vi "Property Dialog.vi"(6 "Control Ref Queue":T29, 7 "Data":refnum<class "3D Plot Datatype.lvclass">[](array[class]), 8 "error in (no error)":errorcluster, 9 "Object Cluster In":T28, 11 "3D Bar in":refnum<class "3D Bar.lvclass">) -> (0 "error out":errorcluster, 1 "Object Cluster Out":T28, 3 "3D Bar out":refnum<class "3D Bar.lvclass">, 4 "Cancel?":bool)   [LabVIEW 2020, in "3D Bar.lvclass"]
uses:
  <vilib>/Math Plots/3D Math Plots/3D Bar/3D Bar/3D Bar.lvclass
  e:/builds/penguin/labview/branches/2020/dev/dist/vi.lib/Math Plots/3D Math Plots/3D Plot/3D Plot/3D Plot.lvclass
  <vilib>/Math Plots/3D Math Plots/3D Plot/Action String/3DMathPlot Ctrl Act Queue.ctl
  <vilib>/Math Plots/3D Math Plots/3D Plot/Action String/3DMathPlot Ctrl Act Cluster.ctl
  <vilib>/Math Plots/3D Math Plots/3D Plot/Action String/3DMathPlot State Class.ctl
  <vilib>/Math Plots/3D Math Plots/3D Plot/3D Plot/Typedef/Object Cluster.ctl
  <vilib>/Math Plots/3D Math Plots/3D Plot/3D Plot Datatype/3D Plot Datatype.lvclass
  <vilib>/Math Plots/3D Math Plots/3D Bar/3D Bar/Typedef/3D Bar Property Array.ctl
  <vilib>/Math Plots/3D Math Plots/3D Bar/3D Bar/Typedef/3D Bar Property.ctl
  <vilib>/Math Plots/3D Math Plots/3D Plot/3D Plot/Typedef/Line Type.ctl
  <vilib>/Math Plots/3D Math Plots/3D Plot/3D Plot/Typedef/Cursor Property Array.ctl
  <vilib>/Math Plots/3D Math Plots/3D Plot/3D Plot/Typedef/Cursor Property.ctl
  <vilib>/Math Plots/3D Math Plots/3D Plot/3D Plot/Typedef/Cursor Position.ctl
  <vilib>/Math Plots/3D Math Plots/3D Plot/3D Plot/Typedef/Cursor Point.ctl
  <vilib>/Math Plots/3D Math Plots/3D Plot/3D Plot/Typedef/Sprite Type.ctl
  <vilib>/Math Plots/3D Math Plots/3D Plot/3D Plot/Typedef/Cursor Line.ctl
  <vilib>/Math Plots/3D Math Plots/3D Plot/3D Plot/Typedef/Cursor Plane.ctl
  <vilib>/Math Plots/3D Math Plots/3D Plot/3D Plot/Typedef/Cursor Text.ctl
  <vilib>/Math Plots/3D Math Plots/3D Plot/3D Plot/Typedef/Format Property.ctl
  <vilib>/Math Plots/3D Math Plots/3D Plot/3D Plot/Typedef/Value Pair Property.ctl
  <vilib>/Math Plots/3D Math Plots/3D Plot/3D Plot/Typedef/Value Pair Cluster.ctl
  <vilib>/Math Plots/3D Math Plots/3D Plot/3D Plot/Typedef/Axis Property.ctl
  <vilib>/Math Plots/3D Math Plots/3D Plot/3D Plot/Typedef/Caption Property.ctl
  <vilib>/Math Plots/3D Math Plots/3D Plot/3D Plot/Typedef/Label Property.ctl
  <vilib>/Math Plots/3D Math Plots/3D Plot/3D Plot/Typedef/Range Property.ctl
  <vilib>/Math Plots/3D Math Plots/3D Plot/3D Plot/Typedef/Range Clusters.ctl
  <vilib>/Math Plots/3D Math Plots/3D Plot/3D Plot/Typedef/Grid Property.ctl
  <vilib>/Math Plots/3D Math Plots/3D Plot/3D Plot/Typedef/Tick Property.ctl
  <vilib>/Math Plots/3D Math Plots/3D Plot/3D Plot/Typedef/Light Property.ctl
  <vilib>/Math Plots/3D Math Plots/3D Plot/3D Plot/Typedef/Light Specific.ctl
  <vilib>/Math Plots/3D Math Plots/3D Plot/3D Plot/Typedef/Graph Property.ctl
  <vilib>/Math Plots/3D Math Plots/3D Plot/3D Plot/Typedef/General Property.ctl
  <vilib>/Math Plots/3D Math Plots/3D Plot/3D Plot/Typedef/View Property.ctl
  <vilib>/Math Plots/3D Math Plots/3D Plot/3D Plot/Typedef/Grid Plane.ctl
  <vilib>/Math Plots/3D Math Plots/3D Plot/3D Plot/Typedef/Temp Scene State.ctl
  <vilib>/Math Plots/3D Math Plots/3D Plot/3D Plot/Typedef/Temp Scene Data Action.ctl
  <vilib>/Math Plots/3D Math Plots/3D Bar/3D Bar/3D Bar.lvclass/3D Bar.ctl
  <vilib>/Math Plots/3D Math Plots/3D Plot/3D Plot/3D Plot.lvclass
panel:
  in  "Graph Property":T1
  in  "Light Property":T5
  in  "Axis Property":T7
  in  "Value Pair Property":T14
  in  "Format Property":T16
  in  "Cursor Property Array":T17
  in  "3D Bar Property Array":T26
  in  "Dialog Tab":enum32{"UI", "Input & Output"}(tab)
  in  "Cancel":bool
  in  "Help":bool
  in  "OK":bool
  in  "Page List":i32(listbox) caption="Page list"
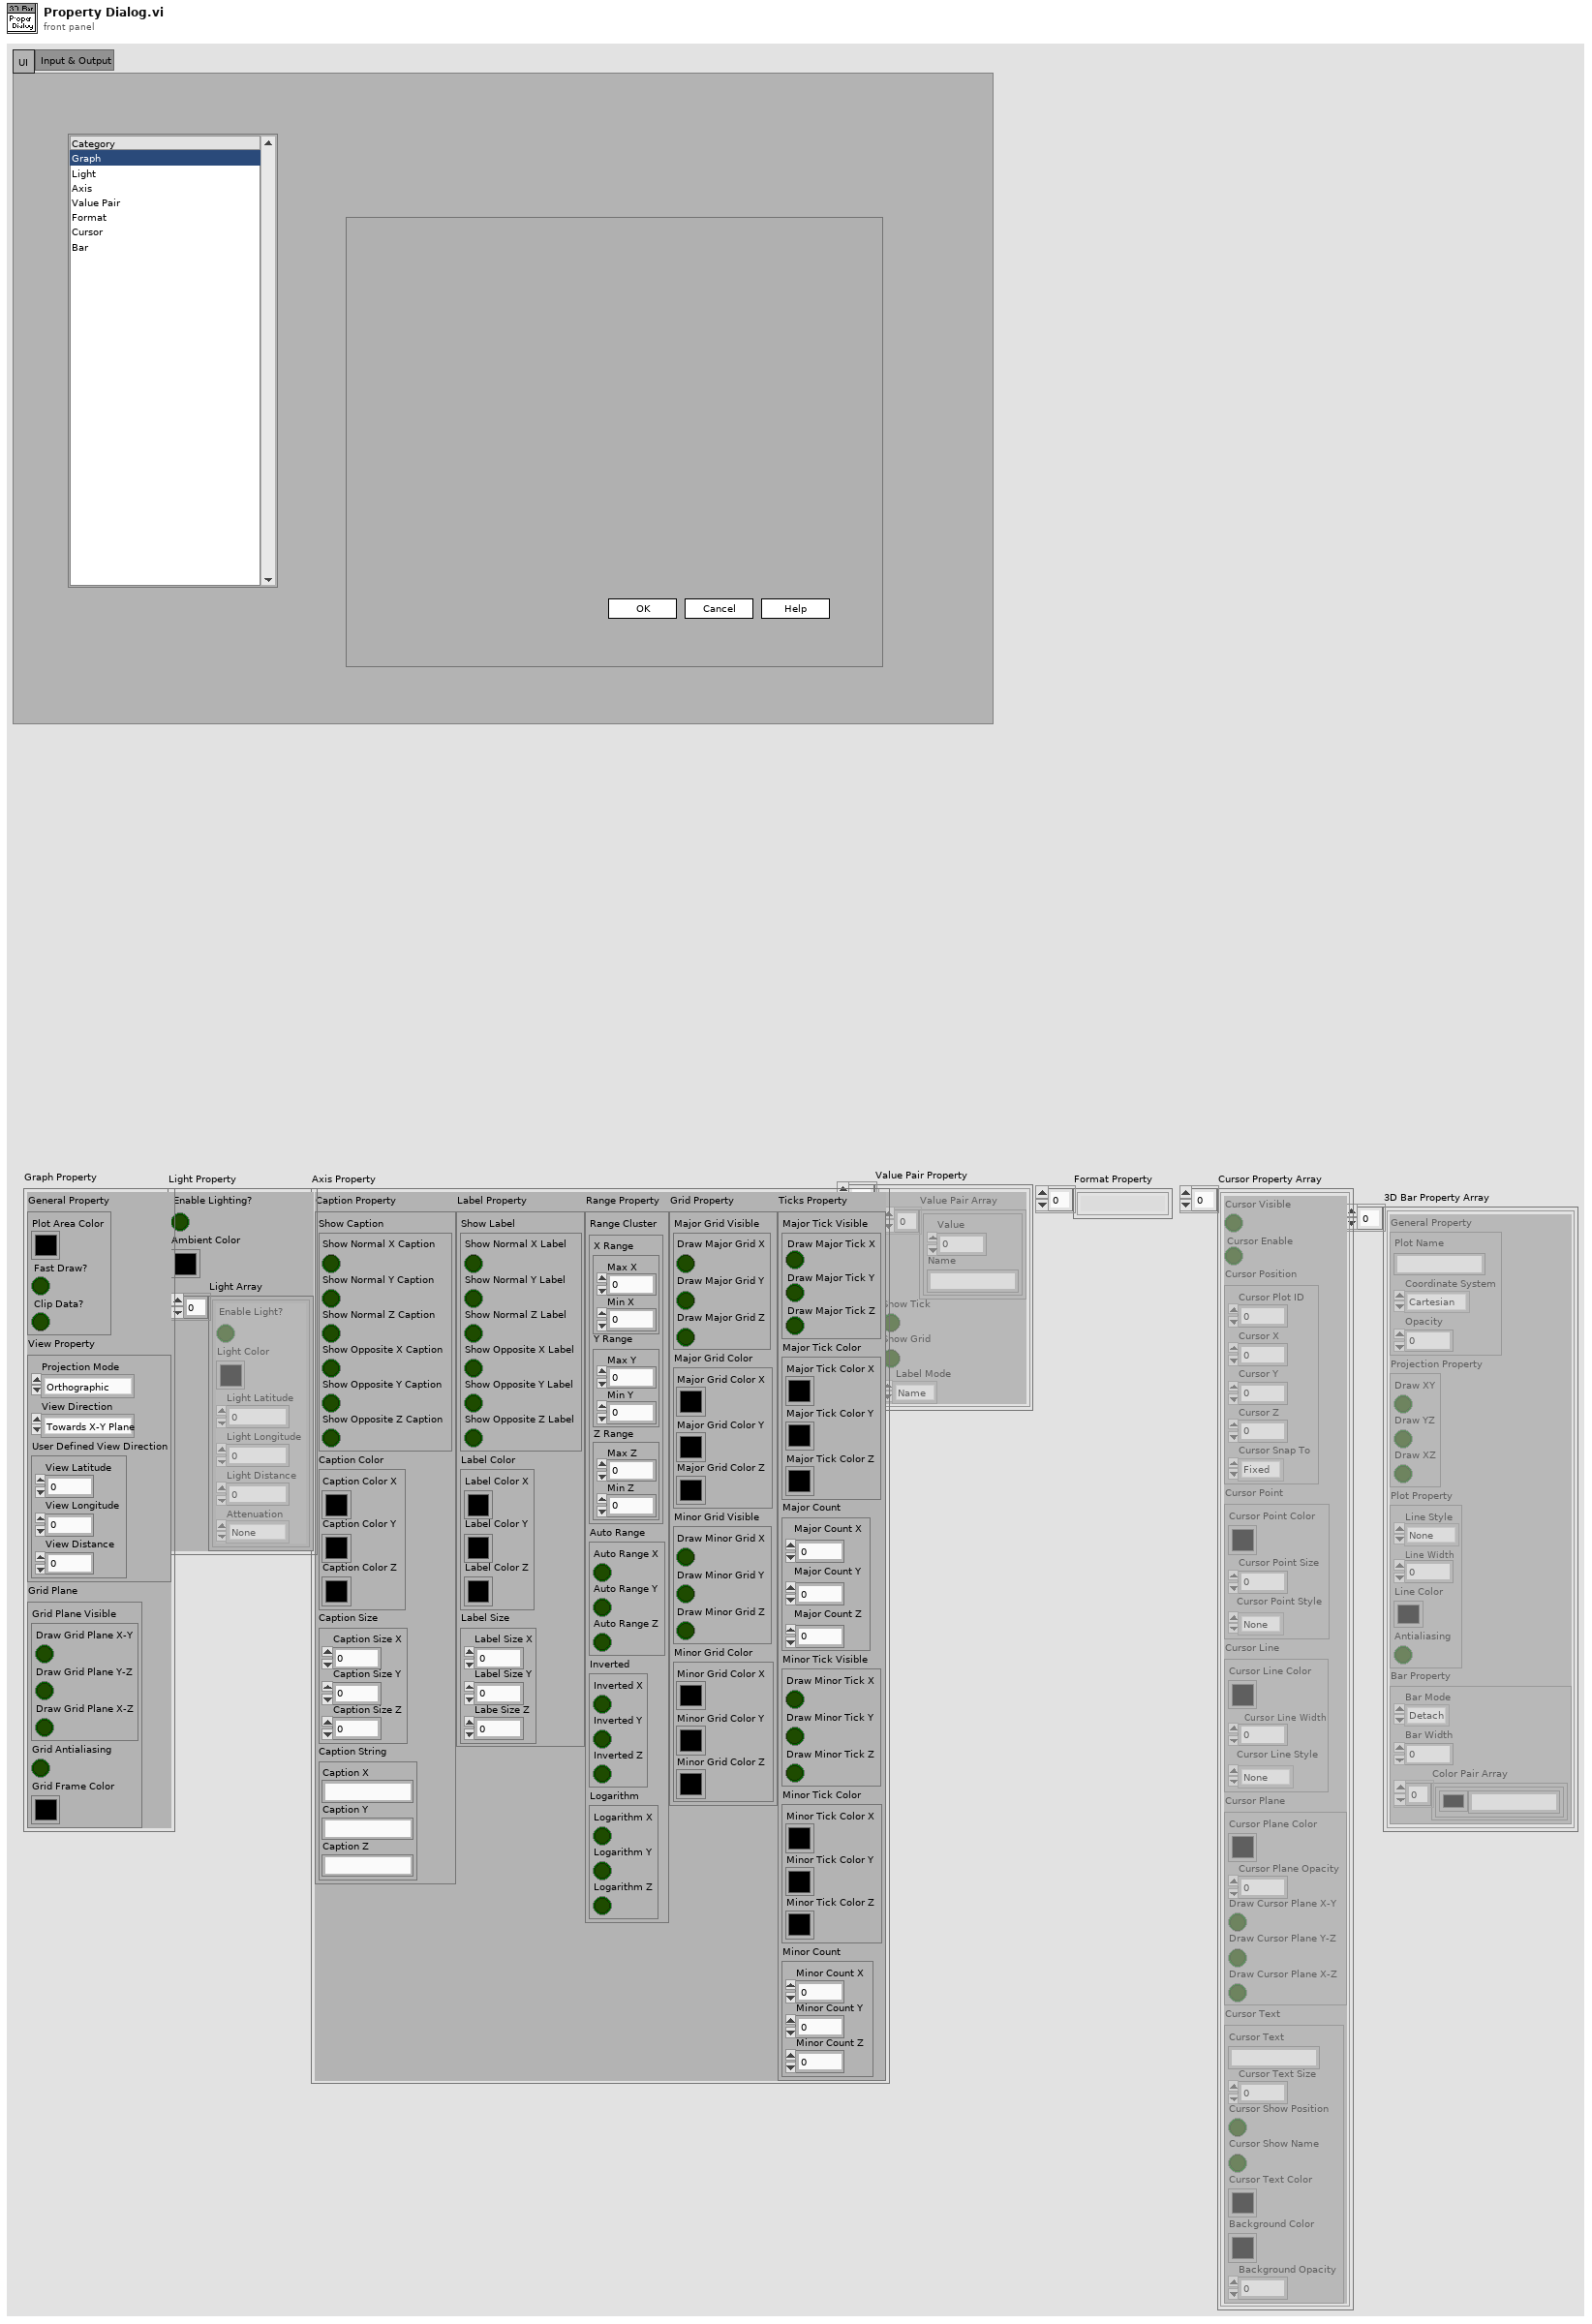
[diagram p1: front panel]
types:
  T1 = typedef "3D Plot.lvclass/Graph Property.ctl" = cluster{"General Property":T2, "View Property":T3, "Grid Plane":T4}
  T2 = typedef "3D Plot.lvclass/General Property.ctl" = cluster{"Plot Area Color":u32, "Fast Draw?":bool, "Clip Data?":bool}
  T3 = typedef "3D Plot.lvclass/View Property.ctl" = cluster{"Projection Mode":enum16{"Orthographic", "Perspective"}, "View Direction":enum32{"Towards X-Y Plane", "Towards X-Z Plane", "Towards Y-Z Plane", "User Defined"}, "User Defined View Direction":cluster{"View Latitude":sgl, "View Longitude":sgl, "View Distance":sgl}}
  T4 = typedef "3D Plot.lvclass/Grid Plane.ctl" = cluster{"Grid Plane Visible":cluster{"Draw Grid Plane X-Y":bool, "Draw Grid Plane Y-Z":bool, "Draw Grid Plane X-Z":bool}, "Grid Antialiasing":bool, "Grid Frame Color":u32}
  T5 = typedef "3D Plot.lvclass/Light Property.ctl" = cluster{"Enable Lighting?":bool, "Ambient Color":u32, "Light Array":T6[]}
  T6 = typedef "3D Plot.lvclass/Light Specific.ctl" = cluster{"Enable Light?":bool, "Light Color":u32, "Light Latitude":sgl, "Light Longitude":sgl, "Light Distance":sgl, "Attenuation":enum16{"None", "Linear", "Quadratic"}}
  T7 = typedef "3D Plot.lvclass/Axis Property.ctl" = cluster{"Caption Property":T8, "Label Property":T9, "Range Property":T10, "Grid Property":T12, "Ticks Property":T13}
  T8 = typedef "3D Plot.lvclass/Caption Property.ctl" = cluster{"Show Caption":cluster{"Show Normal X Caption":bool, "Show Normal Y Caption":bool, "Show Normal Z Caption":bool, "Show Opposite X Caption":bool, "Show Opposite Y Caption":bool, "Show Opposite Z Caption":bool}, "Caption Color":cluster{"Caption Color X":u32, "Caption Color Y":u32, "Caption Color Z":u32}, "Caption Size":cluster{"Caption Size X":u16, "Caption Size Y":u16, "Caption Size Z":u16}, "Caption String":cluster{"Caption X":string, "Caption Y":string, "Caption Z ":string}}
  T9 = typedef "3D Plot.lvclass/Label Property.ctl" = cluster{"Show Label":cluster{"Show Normal X Label":bool, "Show Normal Y Label":bool, "Show Normal Z Label":bool, "Show Opposite X Label":bool, "Show Opposite Y Label":bool, "Show Opposite Z Label":bool}, "Label Color":cluster{"Label Color X":u32, "Label Color Y":u32, "Label Color Z":u32}, "Label Size":cluster{"Label Size X":u16, "Label Size Y":u16, "Labe Size Z":u16}}
  T10 = typedef "3D Plot.lvclass/Range Property.ctl" = cluster{"Range Cluster":T11, "Auto Range":cluster{"Auto Range X":bool, "Auto Range Y":bool, "Auto Range Z":bool}, "Inverted":cluster{"Inverted X":bool, "Inverted Y":bool, "Inverted Z":bool}, "Logarithm":cluster{"Logarithm X":bool, "Logarithm Y":bool, "Logarithm Z":bool}}
  T11 = typedef "3D Plot.lvclass/Range Clusters.ctl" = cluster{"X Range":cluster{"Max X":sgl, "Min X":sgl}, "Y Range":cluster{"Max Y":sgl, "Min Y":sgl}, "Z Range":cluster{"Max Z":sgl, "Min Z":sgl}}
  T12 = typedef "3D Plot.lvclass/Grid Property.ctl" = cluster{"Major Grid Visible":cluster{"Draw Major Grid X":bool, "Draw Major Grid Y":bool, "Draw Major Grid Z":bool}, "Major Grid Color":cluster{"Major Grid Color X":u32, "Major Grid Color Y":u32, "Major Grid Color Z":u32}, "Minor Grid Visible":cluster{"Draw Minor Grid X":bool, "Draw Minor Grid Y":bool, "Draw Minor Grid Z":bool}, "Minor Grid Color":cluster{"Minor Grid Color X":u32, "Minor Grid Color Y":u32, "Minor Grid Color Z":u32}}
  T13 = typedef "3D Plot.lvclass/Tick Property.ctl" = cluster{"Major Tick Visible":cluster{"Draw Major Tick X":bool, "Draw Major Tick Y":bool, "Draw Major Tick Z":bool}, "Major Tick Color":cluster{"Major Tick Color X":u32, "Major Tick Color Y":u32, "Major Tick Color Z":u32}, "Major Count":cluster{"Major Count X":u16, "Major Count Y":u16, "Major Count Z":u16}, "Minor Tick Visible":cluster{"Draw Minor Tick X":bool, "Draw Minor Tick Y":bool, "Draw Minor Tick Z":bool}, "Minor Tick Color":cluster{"Minor Tick Color X":u32, "Minor Tick Color Y":u32, "Minor Tick Color Z":u32}, "Minor Count":cluster{"Minor Count X":u16, "Minor Count Y":u16, "Minor Count Z":u16}}
  T14 = typedef "3D Plot.lvclass/Value Pair Property.ctl" = T15[]
  T15 = typedef "3D Plot.lvclass/Value Pair Cluster.ctl" = cluster{"Value Pair Array":cluster{"Value":sgl, "Name":string}[], "Show Tick":bool, "Show Grid":bool, " Label Mode":enum16{"Name", "Value", "None"}}
  T16 = typedef "3D Plot.lvclass/Format Property.ctl" = string[]
  T17 = typedef "3D Plot.lvclass/Cursor Property Array.ctl" = T18[]
  T18 = typedef "3D Plot.lvclass/Cursor Property.ctl" = cluster{"Cursor Visible":bool, "Cursor Enable":bool, "Cursor Position":T19, "Cursor Point":T20, "Cursor Line":T22, "Cursor Plane":T24, "Cursor Text":T25}
  T19 = typedef "3D Plot.lvclass/Cursor Position.ctl" = cluster{"Cursor Plot ID":i32, "Cursor X":sgl, "Cursor Y":sgl, "Cursor Z":sgl, "Cursor Snap To":enum16{"Fixed", "Nearest Plot", "Snap to Plot"}}
  T20 = typedef "3D Plot.lvclass/Cursor Point.ctl" = cluster{"Cursor Point Color":u32, "Cursor Point Size":sgl, "Cursor Point Style":T21}
  T21 = typedef "3D Plot.lvclass/Sprite Type.ctl" = enum16{"None", "Empty Square", "Solid Square", "Empty Diamond", "Solid Diamond", "Empty Circle", "Solid Circle", "Asterisk", "Bold X", "Wireframe Sphere", "Solid Sphere", "Wireframe Cube", "Solid Cube"}
  T22 = typedef "3D Plot.lvclass/Cursor Line.ctl" = cluster{"Cursor Line Color":u32, "Cursor Line Width":sgl, "Cursor Line Style":T23}
  T23 = typedef "3D Plot.lvclass/Line Type.ctl" = enum16{"None", "Solid", "Dash", "Dot", "Dash Dot"}
  T24 = typedef "3D Plot.lvclass/Cursor Plane.ctl" = cluster{"Cursor Plane Color":u32, "Cursor Plane Opacity":sgl, "Draw Cursor Plane X-Z":bool, "Draw Cursor Plane Y-Z":bool, "Draw Cursor Plane X-Y":bool}
  T25 = typedef "3D Plot.lvclass/Cursor Text.ctl" = cluster{"Cursor Text":string, "Cursor Text Size":u16, "Cursor Show Position":bool, "Cursor Show Name":bool, "Cursor Text Color":u32, "Background Color":u32, "Background Opacity":sgl}
  T26 = typedef "3D Bar.lvclass/3D Bar Property Array.ctl" = T27[]
  T27 = typedef "3D Bar.lvclass/3D Bar Property.ctl" = cluster{"General Property":cluster{"Plot Name":string, "Coordinate System":enum16{"Cartesian", "Cylindrical", "Spherical"}, "Opacity":sgl}, "Projection Property":cluster{"Draw XY":bool, "Draw YZ":bool, "Draw XZ":bool}, "Plot Property":cluster{"Line Style":T23, "Line Width":sgl, "Line Color":u32, "Antialiasing":bool}, "Bar Property":cluster{"Bar Mode":enum16{"Detach", "Group", "Stack"}, "Bar Width":sgl, "Color Pair Array":cluster{"Color":u32, "String":string}[]}}
  T28 = typedef "3D Plot.lvclass/Object Cluster.ctl" = cluster{"Root Scene Object":refnum<vi>, "Fast Root Scene Object":refnum<vi>}
  T29 = typedef "3DMathPlot Ctrl Act Queue.ctl" = refnum<queue>
  T30 = typedef "3D Plot.lvclass/Temp Scene State.ctl" = enum16{"Create", "Update Scene", "Get Plot Representation", "Destory"}
  T31 = typedef "3D Plot.lvclass/Temp Scene Data Action.ctl" = enum16{"Data Class", "Property Class", "Object Cluster", "Control Queue"}
  T32 = typedef "3D Plot.lvclass/Property Cluster.ctl" = cluster{"Graph Property":T1, "Light Property":T5, "Axis Property":T7, "Value Pair Property":T14, "Format Property":T16, "Cursor Property Array":T17, "Appearance Property":T33}
  T33 = typedef "3D Plot.lvclass/Apearance Property.ctl" = cluster{"Visibility":T34, "Active Index":cluster{"Active Plot":i32, "Active Cursor":i32, "Active Axis":enum16{"X-axis", "Y-axis", "Z-axis"}, "Active Value Pair":enum16{"X-axis", "Y-axis", "Z-axis"}, "Active Light":enum16{"Light 0", "Light 1", "Light 2", "Light 3"}}, "Backup Data":cluster{"Plot Name":string[]}}
  T34 = typedef "3D Plot.lvclass/Item Visibility.ctl" = cluster{"Projection Palette":bool, "Color Ramp Palette":bool}
  T35 = enum32{"Bad", "Idle", "Run top level", "Running"}[]
  T36 = enum32{"Bad", "Idle", "Run top level", "Running"}
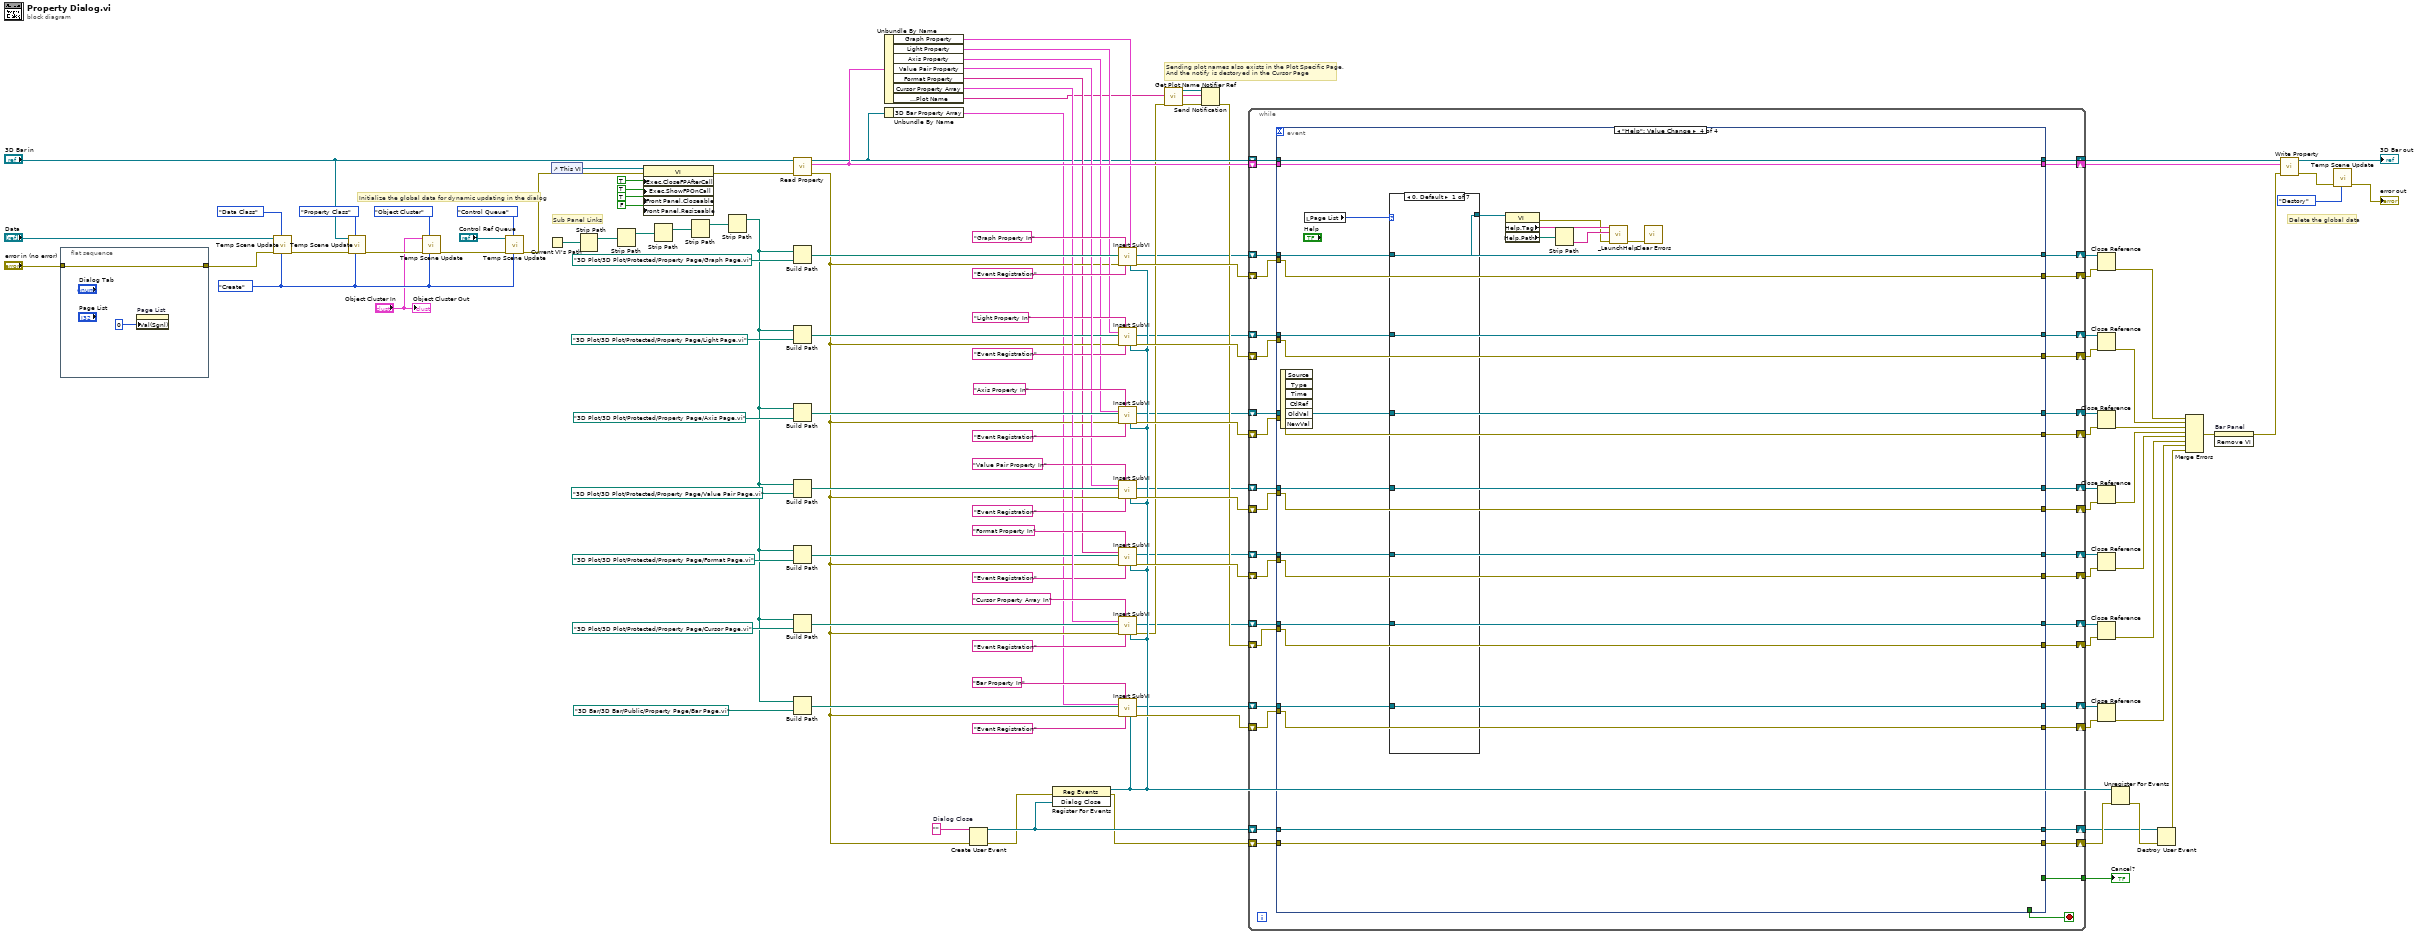
[diagram p0: block diagram]
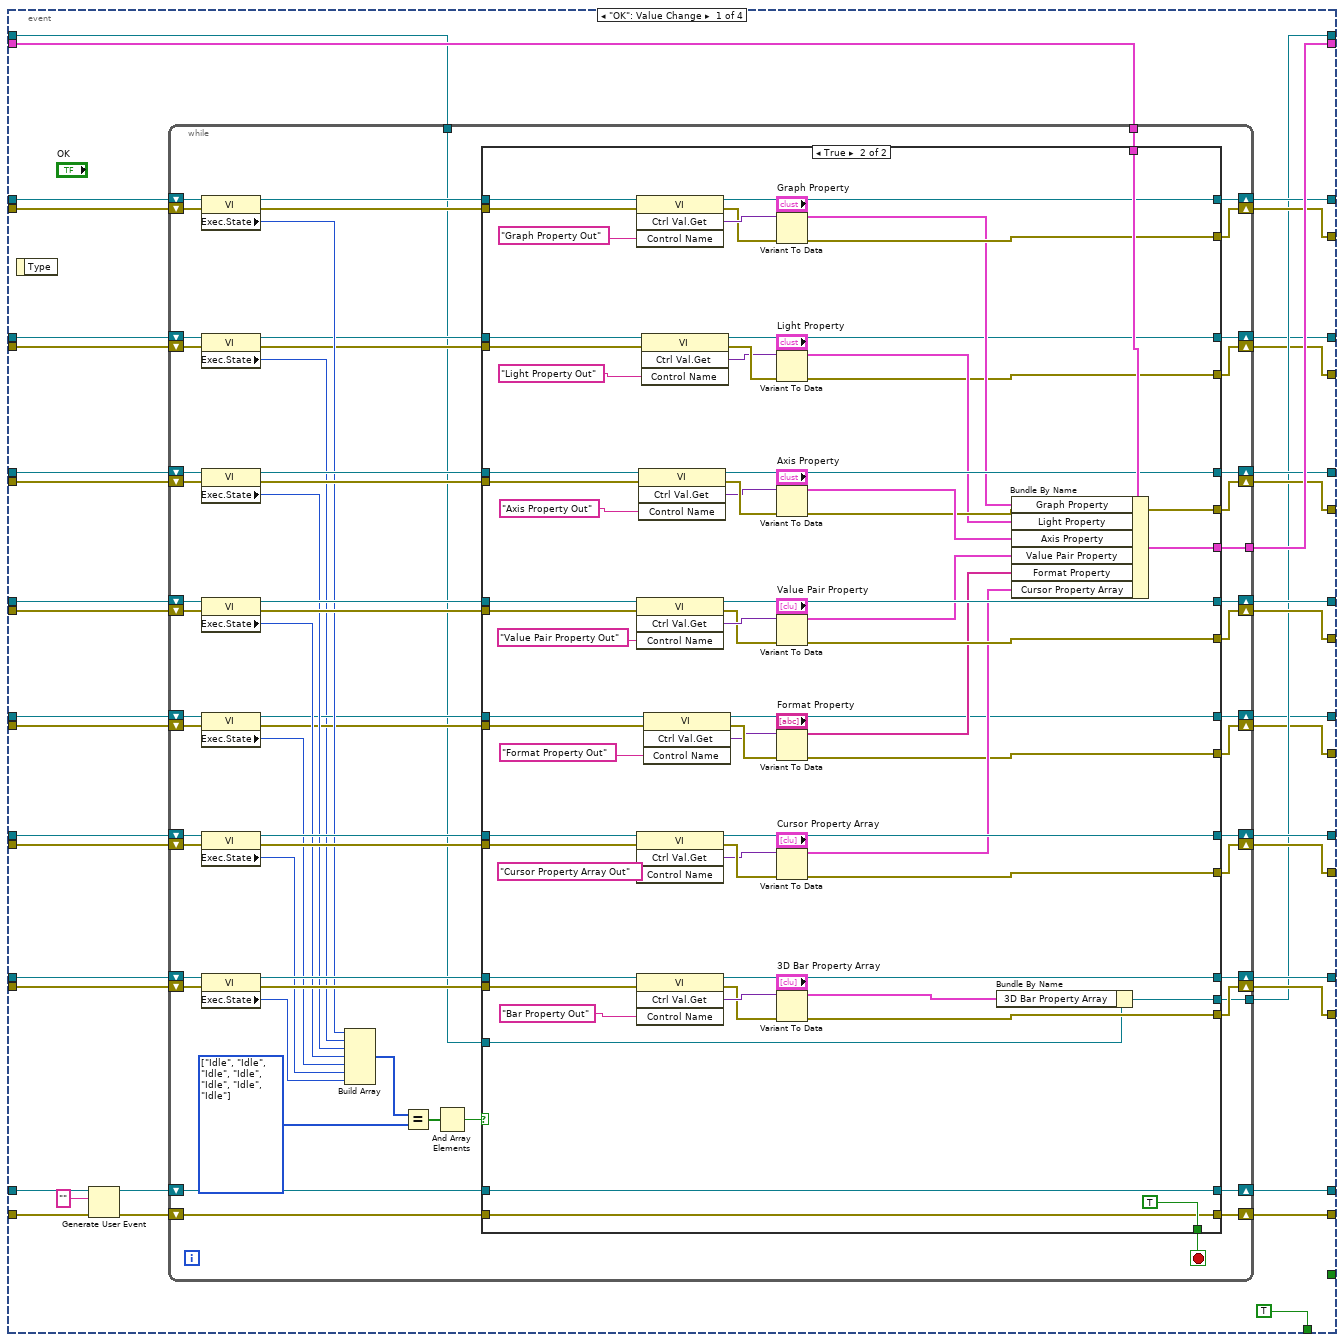
[diagram p2: hidden frame]
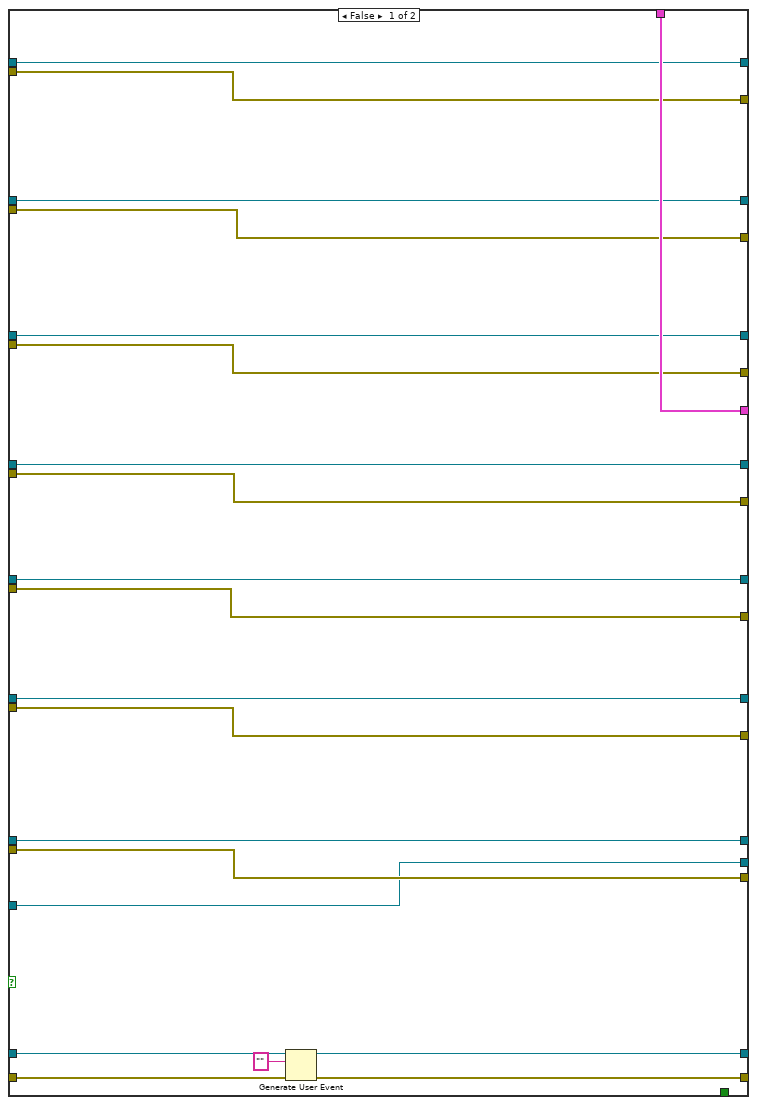
[diagram p3: hidden frame]
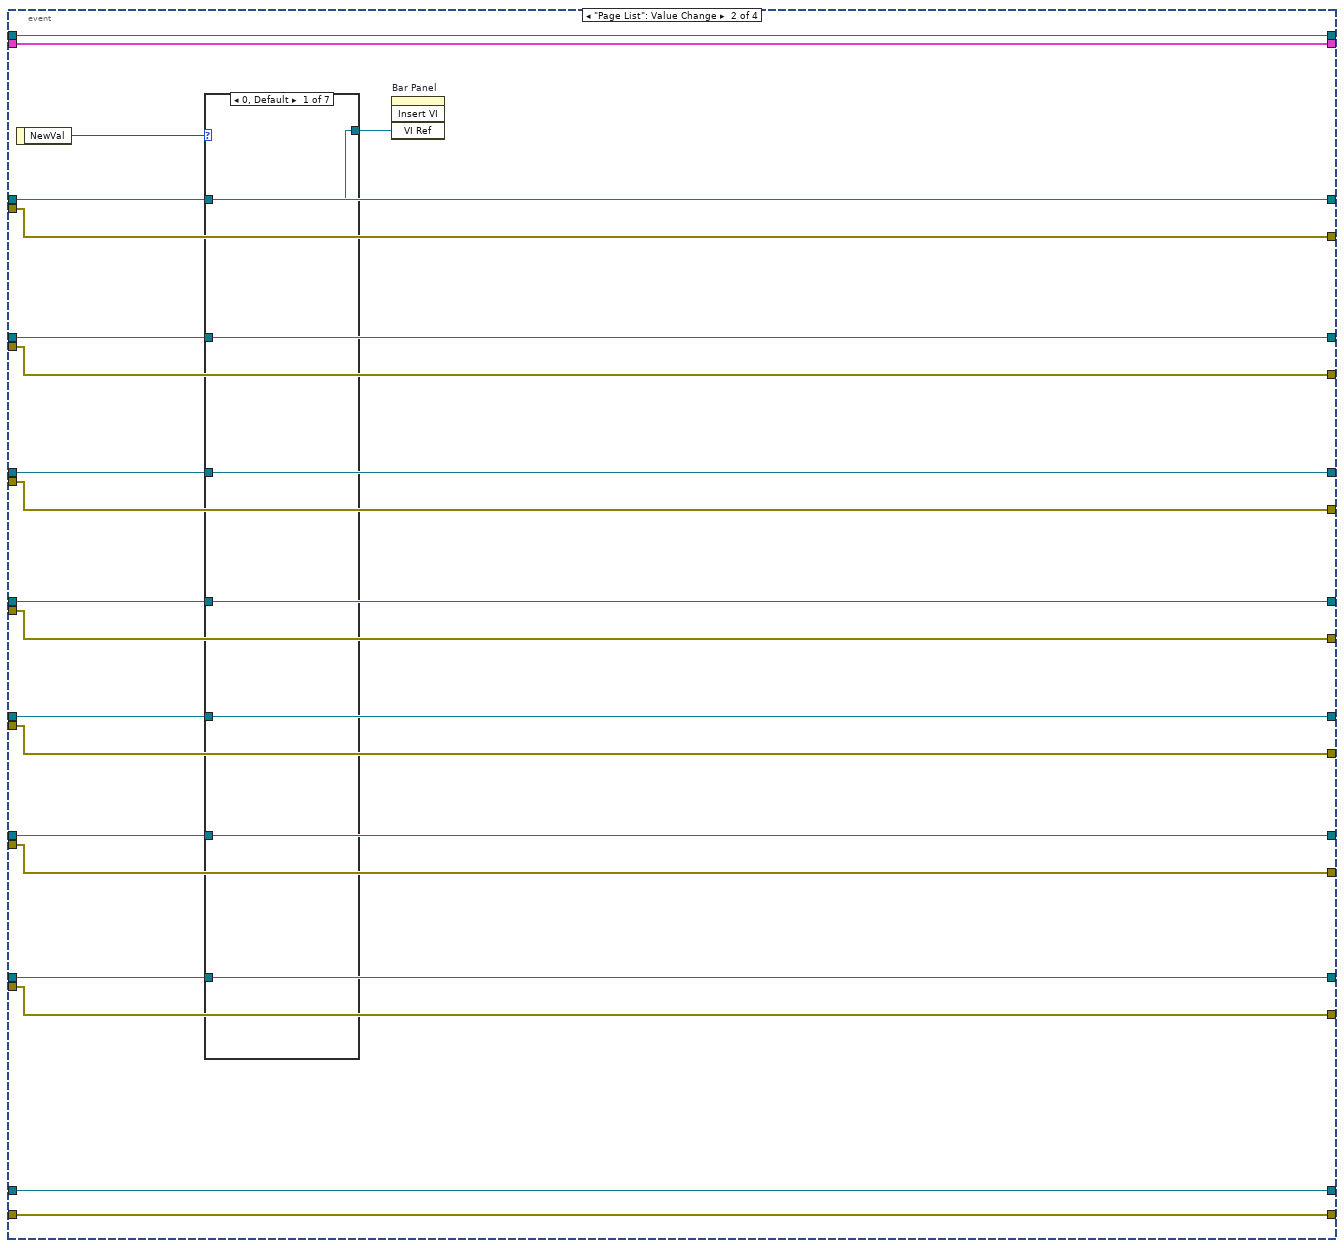
[diagram p4: hidden frame]
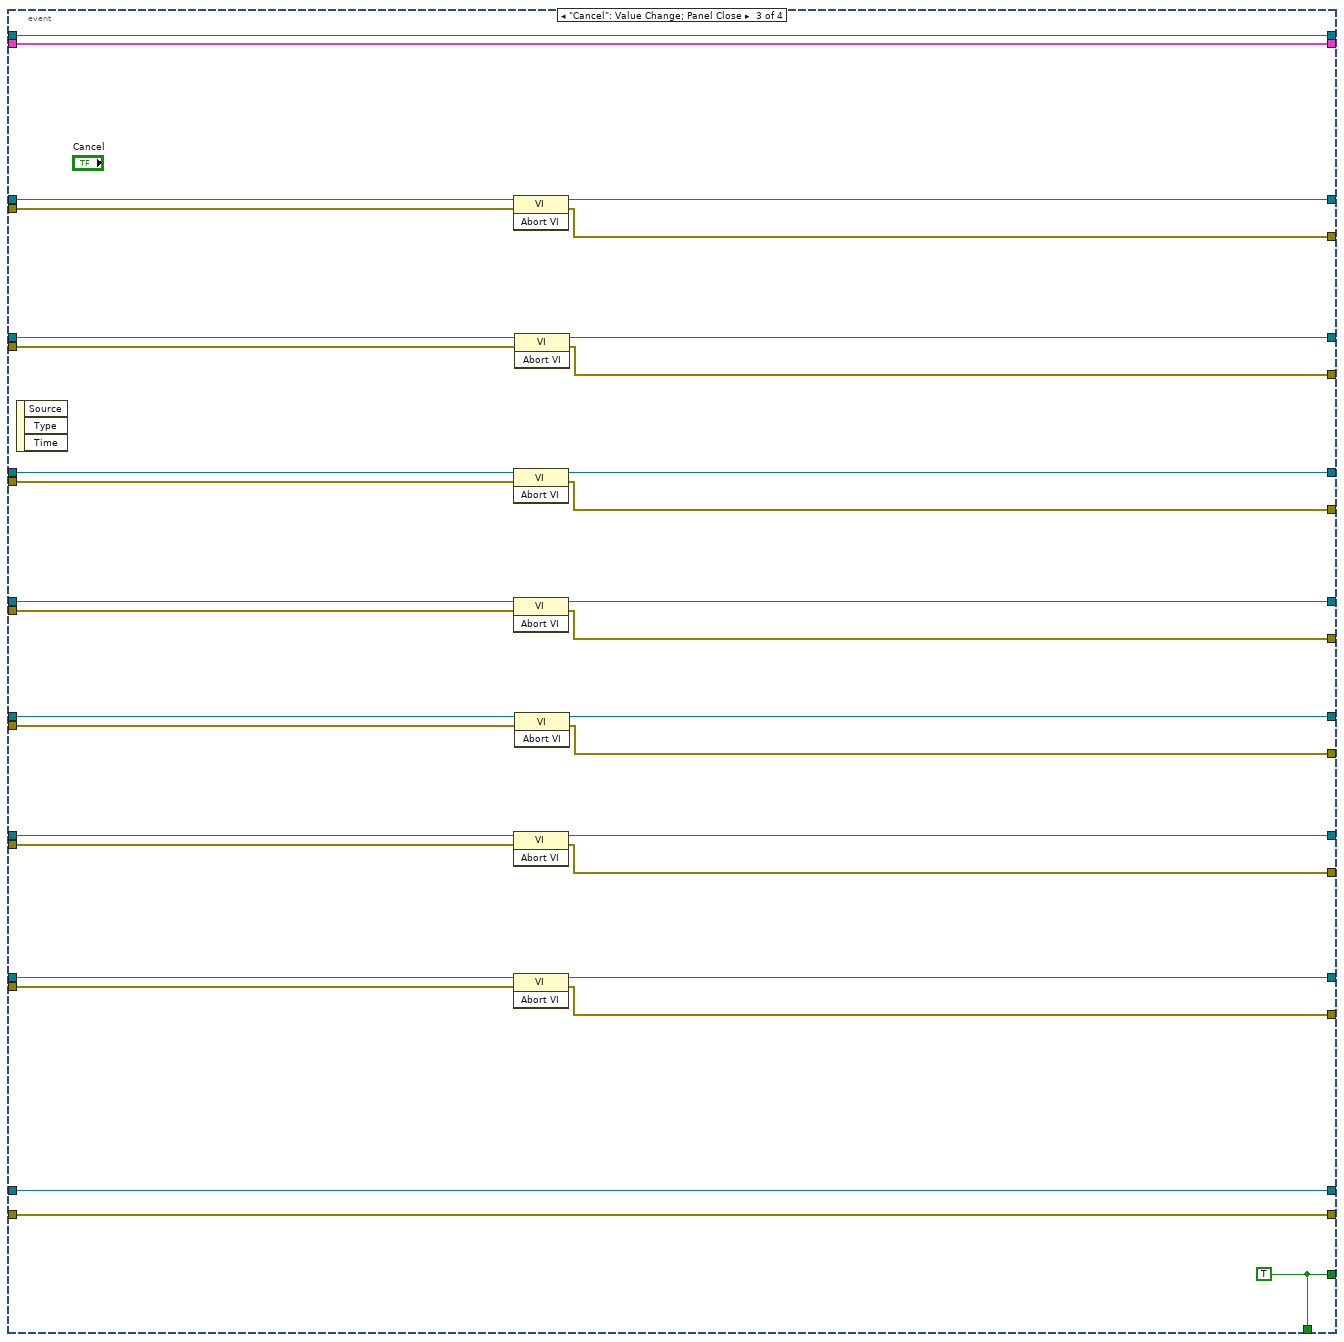
[diagram p11: hidden frame]
diagram:
  w36 = Temp_Scene_State."Create" ("State")
  w113 = ""  # Dialog Close
  # "Sending plot names also exists in the Plot Specific Page,\nAnd the notify is destoryed in the Cursor Page"
  # "Delete the global data"
  # "Initialize the global data for dynamic updating in the dialog"
  # "Sub Panel Links"
  n1 = flat-sequence {
    tunnel: [w124] -> w35
    tunnel: "error in (no error)" -> [w124]
    frame #0 {
      n2 = property on="Page List" class="LstBox (strict)"("Val(Sgnl)"=0) -> ()  [unwired: 2 in, 2 out]
    }
  }
  n3 = call <vilib>:"Temp Scene Update.vi"("State"=w36, "Data Name"=Temp_Scene_Data_Action."Data Class", "error in (no error)"=w35, "Property In"="Data") -> ("error out"=w48:errorcluster)  [unwired: 2 in, 5 out]
  n4 = call <vilib>:"Temp Scene Update.vi"("State"=w36, "Data Name"=Temp_Scene_Data_Action."Property Class", "error in (no error)"=w48, "Property In"="3D Bar in") -> ("error out"=w45:errorcluster)  [unwired: 2 in, 5 out]
  n5 = call <vilib>:"Temp Scene Update.vi"("State"=w36, "Data Name"=Temp_Scene_Data_Action."Object Cluster", "error in (no error)"=w45, "Property In"="Object Cluster In") -> ("error out"=w46:errorcluster)  [unwired: 2 in, 5 out]
  n6 = call <vilib>:"Temp Scene Update.vi"("State"=w36, "Data Name"=Temp_Scene_Data_Action."Control Queue", "error in (no error)"=w46, "Property In"="Control Ref Queue") -> ("error out"=w40:errorcluster)  [unwired: 2 in, 5 out]
  n7 = Current VI's Path() -> (path=w121:path)
  n8 = control-ref of="This VI"() -> (w82:refnum<vi>)
  n9 = Strip Path(path=w121) -> (stripped path=w120:path)  [unwired: 1 out]
  n10 = Strip Path(path=w120) -> (stripped path=w115:path)  [unwired: 1 out]
  n11 = property class="VI"(reference=w82, error in=w40, "Exec.CloseFPAfterCall"=TRUE ("Execution:Close After Call"), "Exec.ShowFPOnCall"=TRUE ("Execution:Show Front Panel On Call"), "Front Panel.Closeable"=TRUE ("Front Panel Window:Closeable"), "Front Panel.Resizeable"=FALSE ("Front Panel Window:Resizeable")) -> (error out=w81:errorcluster)  [unwired: 1 out]
  n12 = Strip Path(path=w115) -> (stripped path=w80:path)  [unwired: 1 out]
  n13 = Strip Path(path=w80) -> (stripped path=w29:path)  [unwired: 1 out]
  n14 = Strip Path(path=w29) -> (stripped path=w28:path)  [unwired: 1 out]
  n15 = call <vilib>:"Read Property.vi"("error in (no error)"=w81, "3D Plot.lvclass in"="3D Bar in") -> ("error out"=w56:errorcluster, "Property Cluster"=w117:T32, "3D Plot.lvclass out"=w52:refnum<class "3D Bar.lvclass">)  [unwired: 7 out]
  n16 = Build Path(base path=w28, name or relative path=path "3D Plot/3D Plot/Protected/Property Page/Graph Page.vi") -> (appended path=w119:path)
  n17 = Build Path(base path=w28, name or relative path=path "3D Plot/3D Plot/Protected/Property Page/Light Page.vi") -> (appended path=w69:path)
  n18 = Build Path(base path=w28, name or relative path=path "3D Plot/3D Plot/Protected/Property Page/Axis Page.vi") -> (appended path=w109:path)
  n19 = Build Path(base path=w28, name or relative path=path "3D Plot/3D Plot/Protected/Property Page/Value Pair Page.vi") -> (appended path=w102:path)
  n20 = Build Path(base path=w28, name or relative path=path "3D Plot/3D Plot/Protected/Property Page/Format Page.vi") -> (appended path=w59:path)
  n21 = Build Path(base path=w28, name or relative path=path "3D Plot/3D Plot/Protected/Property Page/Cursor Page.vi") -> (appended path=w96:path)
  n22 = Build Path(base path=w28, name or relative path=path "3D Bar/3D Bar/Public/Property Page/Bar Page.vi") -> (appended path=w89:path)
  n23 = Unbundle By Name(w117) -> ("Graph Property"=w73:T1, "Light Property"=w64:T5, "Axis Property"=w68:T7, "Value Pair Property"=w101:T14, "Format Property"=w55:T16, "Cursor Property Array"=w94:T17, "Appearance Property.Backup Data.Plot Name"=w25:string[])
  n24 = Unbundle By Name(w52) -> ("3D Bar Property Array"=w51:T26)
  n25 = Create User Event(user event datatype=w113, error in=w56) -> (user event=w114:refnum<user-event>, error out=w66:errorcluster)
  n26 = register-events(error in=w66, w114) -> (reference out=w30:refnum<event-registration>, error out=w65:errorcluster)  [unwired: 1 in]
  n27 = call <vilib>:"Insert SubVI.vi"("Value 2"=w30, "Value 1"=w73, "Label 2"="Event Registration", "Label 1"="Graph Property In", "error in (no error)"=w56, "VI Path"=w119) -> ("error out"=w118:errorcluster, "vi reference"=w21:refnum<vi>)  [unwired: 3 in, 1 out]
  n28 = call <vilib>:"Insert SubVI.vi"("Value 2"=w30, "Value 1"=w64, "Label 2"="Event Registration", "Label 1"="Light Property In", "error in (no error)"=w56, "VI Path"=w69) -> ("error out"=w67:errorcluster, "vi reference"=w20:refnum<vi>)  [unwired: 3 in, 1 out]
  n29 = call <vilib>:"Insert SubVI.vi"("Value 2"=w30, "Value 1"=w68, "Label 2"="Event Registration", "Label 1"="Axis Property In", "error in (no error)"=w56, "VI Path"=w109) -> ("error out"=w106:errorcluster, "vi reference"=w19:refnum<vi>)  [unwired: 3 in, 1 out]
  n30 = call <vilib>:"Insert SubVI.vi"("Value 2"=w30, "Value 1"=w101, "Label 2"="Event Registration", "Label 1"="Value Pair Property In", "error in (no error)"=w56, "VI Path"=w102) -> ("error out"=w99:errorcluster, "vi reference"=w18:refnum<vi>)  [unwired: 3 in, 1 out]
  n31 = call <vilib>:"Insert SubVI.vi"("Value 2"=w30, "Value 1"=w55, "Label 2"="Event Registration", "Label 1"="Format Property In", "error in (no error)"=w56, "VI Path"=w59) -> ("error out"=w54:errorcluster, "vi reference"=w17:refnum<vi>)  [unwired: 3 in, 1 out]
  n32 = call <vilib>:"Insert SubVI.vi"("Value 2"=w30, "Value 1"=w94, "Label 2"="Event Registration", "Label 1"="Cursor Property Array In", "error in (no error)"=w56, "VI Path"=w96) -> ("error out"=w24:errorcluster, "vi reference"=w16:refnum<vi>)  [unwired: 3 in, 1 out]
  n33 = call <vilib>:"Insert SubVI.vi"("Value 2"=w30, "Value 1"=w51, "Label 2"="Event Registration", "Label 1"="Bar Property In", "error in (no error)"=w56, "VI Path"=w89) -> ("error out"=w91:errorcluster, "vi reference"=w15:refnum<vi>)  [unwired: 3 in, 1 out]
  n34 = call <vilib>:"Get Plot Name Notifier Ref.vi"("error in (no error)"=w24) -> ("error out"=w27:errorcluster, "Plot Names Notifier Ref"=w26:refnum<notifier>)  [unwired: 9 out]
  n35 = Send Notification(notification=w25, notifier=w26, error in (no error)=w27) -> (error out=w23:errorcluster)  [unwired: 1 out]
  n36 = while {
    shift-right: [w156] -> w9
    shift-left: w118 -> [w159]
    shift-right: [w157] -> w112
    shift-left: w21 -> [w160]
    shift-right: [w153] -> w7
    shift-left: w106 -> [w151]
    shift-right: [w148] -> w6
    shift-left: w99 -> [w147]
    shift-right: [w145] -> w4
    shift-left: w23 -> [w143]
    shift-right: [w140] -> w3
    shift-left: w91 -> [w141]
    shift-right: [w137] -> w88
    shift-left: w52 -> [w138]
    shift-right: [w161] -> w116
    shift-left: w117 -> [w162]
    tunnel: [w136] -> w79
    shift-right: [w132] -> w63
    shift-left: w20 -> [w134]
    shift-right: [w130] -> w32
    shift-left: w65 -> [w135]
    shift-right: [w131] -> w8
    shift-left: w67 -> [w133]
    shift-right: [w126] -> w5
    shift-left: w54 -> [w128]
    shift-right: [w152] -> w105
    shift-left: w19 -> [w154]
    shift-right: [w149] -> w100
    shift-left: w18 -> [w150]
    shift-right: [w127] -> w53
    shift-left: w17 -> [w129]
    shift-right: [w144] -> w95
    shift-left: w16 -> [w146]
    shift-right: [w139] -> w90
    shift-left: w15 -> [w142]
    shift-right: [w125] -> w31
    shift-left: w114 -> [w155]
    stop <- w158 stop-if-true
    n37 = event shown="[3] \"Help\": Value Change" {
      selector: _ -> [_ _ _ _]
      dyn-events: _ -> [_ _ _ _]
      timeout: _ -> [_ _ _ _]
      tunnel: w162 -> [w202 w374 w415 w440]
      tunnel: [w201 w374 w415 w440] -> w161
      tunnel: w160 -> [w180 w363 w396 w424]
      tunnel: w159 -> [w195 w373 w397 w439]
      tunnel: [TRUE _ w383 _] -> w158
      tunnel: [w199 w363 w394 w424] -> w157
      tunnel: [w198 w373 w395 w439] -> w156
      tunnel: w155 -> [w179 w365 w384 w430]
      tunnel: w154 -> [w181 w361 w401 w421]
      tunnel: [w196 w372 w399 w438] -> w153
      tunnel: [w194 w361 w398 w421] -> w152
      tunnel: w151 -> [w182 w372 w400 w438]
      tunnel: w150 -> [w184 w360 w411 w420]
      tunnel: w147 -> [w183 w371 w413 w437]
      tunnel: [w193 w360 w410 w420] -> w149
      tunnel: [w192 w371 w412 w437] -> w148
      tunnel: w143 -> [w185 w370 w409 w436]
      tunnel: w146 -> [w186 w358 w407 w418]
      tunnel: [w190 w358 w406 w418] -> w144
      tunnel: [w191 w370 w408 w436] -> w145
      tunnel: w142 -> [w178 w357 w403 w417]
      tunnel: w141 -> [w176 w369 w405 w435]
      tunnel: [w189 w369 w404 w435] -> w140
      tunnel: [w188 w357 w402 w417] -> w139
      tunnel: w138 -> [w164 w375 w414 w434]
      tunnel: [w187 w375 w414 w434] -> w137
      tunnel: [_ _ w383 _] -> w136
      tunnel: w135 -> [w175 w366 w389 w431]
      tunnel: w134 -> [w174 w362 w393 w422]
      tunnel: w133 -> [w173 w367 w392 w433]
      tunnel: [w172 w362 w385 w422] -> w132
      tunnel: [w171 w367 w386 w433] -> w131
      tunnel: [w169 w366 w389 w431] -> w130
      tunnel: w129 -> [w168 w359 w391 w419]
      tunnel: w128 -> [w167 w368 w390 w432]
      tunnel: [w166 w368 w387 w432] -> w126
      tunnel: [w165 w359 w388 w419] -> w127
      tunnel: [w163 w365 w384 w430] -> w125
      event "OK": Value Change {
        n38 = event-data() -> ()  [unwired: 2 out]
        n39 = Generate User Event(user event=w179, event data cluster="" ("event data"), error in=w175) -> (user event out=w177:refnum<user-event>, error out=w170:errorcluster)  [unwired: 1 in]
        n40 = while {
          tunnel: w202 -> [w264]
          tunnel: [w263] -> w201
          tunnel: [w228] -> w187
          shift-right: [w220] -> w163
          shift-left: w177 -> [w221]
          tunnel: w164 -> [w203]
          shift-right: [w262] -> w199
          shift-left: w180 -> [w260]
          shift-right: [w261] -> w198
          shift-left: w195 -> [w258]
          shift-right: [w215] -> w172
          shift-left: w174 -> [w218]
          shift-right: [w214] -> w171
          shift-left: w173 -> [w219]
          shift-right: [w247] -> w194
          shift-left: w181 -> [w251]
          shift-right: [w248] -> w196
          shift-left: w182 -> [w246]
          shift-right: [w241] -> w193
          shift-left: w184 -> [w245]
          shift-right: [w240] -> w192
          shift-left: w183 -> [w244]
          shift-right: [w206] -> w165
          shift-left: w168 -> [w211]
          shift-right: [w207] -> w166
          shift-left: w167 -> [w210]
          shift-right: [w238] -> w190
          shift-left: w186 -> [w227]
          shift-right: [w239] -> w191
          shift-left: w185 -> [w235]
          shift-right: [w229] -> w188
          shift-left: w178 -> [w232]
          shift-right: [w230] -> w189
          shift-left: w176 -> [w234]
          shift-right: [w212] -> w169
          shift-left: w170 -> [w213]
          stop <- w252 stop-if-true
          w255 = T35 [enum."Idle", enum."Idle", enum."Idle", enum."Idle", enum."Idle", enum."Idle", enum."Idle"] items=["Bad", "Idle", "Run top level", "Running"]
          n41 = property class="VI"(reference=w260, error in=w258) -> (reference out=w259:refnum<vi>, error out=w257:errorcluster, "Exec.State"=w226:T36)
          n42 = property class="VI"(reference=w218, error in=w219) -> (reference out=w217:refnum<vi>, error out=w216:errorcluster, "Exec.State"=w205:T36)
          n43 = property class="VI"(reference=w251, error in=w246) -> (reference out=w250:refnum<vi>, error out=w249:errorcluster, "Exec.State"=w225:T36)
          n44 = property class="VI"(reference=w245, error in=w244) -> (reference out=w243:refnum<vi>, error out=w242:errorcluster, "Exec.State"=w224:T36)
          n45 = property class="VI"(reference=w211, error in=w210) -> (reference out=w209:refnum<vi>, error out=w208:errorcluster, "Exec.State"=w204:T36)
          n46 = property class="VI"(reference=w227, error in=w235) -> (reference out=w236:refnum<vi>, error out=w237:errorcluster, "Exec.State"=w223:T36)
          n47 = property class="VI"(reference=w232, error in=w234) -> (reference out=w231:refnum<vi>, error out=w233:errorcluster, "Exec.State"=w222:T36)
          n48 = Build Array(w226, w205, w225, w224, w204, w223, w222) -> (w256:T35)
          n49 = Equal?(x=w256, y=w255) -> (x = y?=w254:bool[])
          n50 = And Array Elements(Boolean array=w254) -> (logical AND=w253:bool)
          n51 = case shown="True" w253 {
            tunnel: w264 -> [w285 w355]
            tunnel: [w285 w354] -> w263
            tunnel: [w284 w350] -> w262
            tunnel: [w283 w349] -> w261
            tunnel: w259 -> [w284 w348]
            tunnel: w257 -> [w283 w347]
            tunnel: [_ TRUE] -> w252
            tunnel: w250 -> [w281 w341]
            tunnel: w249 -> [w282 w342]
            tunnel: [w282 w339] -> w248
            tunnel: [w281 w338] -> w247
            tunnel: w243 -> [w279 w334]
            tunnel: w242 -> [w280 w333]
            tunnel: [w279 w332] -> w241
            tunnel: [w280 w331] -> w240
            tunnel: w236 -> [w278 w326]
            tunnel: w237 -> [w277 w327]
            tunnel: [w278 w328] -> w238
            tunnel: [w277 w329] -> w239
            tunnel: w231 -> [w276 w318]
            tunnel: w233 -> [w270 w317]
            tunnel: [w270 w316] -> w230
            tunnel: [w276 w315] -> w229
            tunnel: [w265 w286] -> w228
            tunnel: w221 -> [w275 w314]
            tunnel: [w274 w314] -> w220
            tunnel: w217 -> [w272 w310]
            tunnel: w216 -> [w271 w309]
            tunnel: [w272 w306] -> w215
            tunnel: [w271 w305] -> w214
            tunnel: w213 -> [w269 w304]
            tunnel: [w268 w304] -> w212
            tunnel: w209 -> [w267 w300]
            tunnel: w208 -> [w266 w299]
            tunnel: [w266 w297] -> w207
            tunnel: [w267 w296] -> w206
            tunnel: w203 -> [w265 w288]
            frame False {
              n52 = Generate User Event(user event=w275, event data cluster="" ("event data"), error in=w269) -> (user event out=w274:refnum<user-event>, error out=w268:errorcluster)  [unwired: 1 in]
            }
            frame True {
              n53 = invoke class="VI" method="Ctrl Val.Get"(reference=w348, error in=w347, "Control Name"="Graph Property Out") -> (reference out=w350:refnum<vi>, error out=w351:errorcluster, "Get Control Value Variant"=w352:variant)  [unwired: 1 in, 1 out]
              n54 = invoke class="VI" method="Ctrl Val.Get"(reference=w334, error in=w333, "Control Name"="Value Pair Property Out") -> (reference out=w332:refnum<vi>, error out=w335:errorcluster, "Get Control Value Variant"=w336:variant)  [unwired: 1 in, 1 out]
              n55 = invoke class="VI" method="Ctrl Val.Get"(reference=w326, error in=w327, "Control Name"="Cursor Property Array Out") -> (reference out=w328:refnum<vi>, error out=w325:errorcluster, "Get Control Value Variant"=w324:variant)  [unwired: 1 in, 1 out]
              n56 = invoke class="VI" method="Ctrl Val.Get"(reference=w318, error in=w317, "Control Name"="Bar Property Out") -> (reference out=w315:refnum<vi>, error out=w319:errorcluster, "Get Control Value Variant"=w320:variant)  [unwired: 1 in, 1 out]
              n57 = invoke class="VI" method="Ctrl Val.Get"(reference=w341, error in=w342, "Control Name"="Axis Property Out") -> (reference out=w338:refnum<vi>, error out=w345:errorcluster, "Get Control Value Variant"=w344:variant)  [unwired: 1 in, 1 out]
              n58 = invoke class="VI" method="Ctrl Val.Get"(reference=w310, error in=w309, "Control Name"="Light Property Out") -> (reference out=w306:refnum<vi>, error out=w313:errorcluster, "Get Control Value Variant"=w312:variant)  [unwired: 1 in, 1 out]
              n59 = invoke class="VI" method="Ctrl Val.Get"(reference=w300, error in=w299, "Control Name"="Format Property Out") -> (reference out=w296:refnum<vi>, error out=w303:errorcluster, "Get Control Value Variant"=w302:variant)  [unwired: 1 in, 1 out]
              n60 = Variant To Data(error in=w351, type="Graph Property", Variant=w352) -> (data=w308:T1, error out=w349:errorcluster)
              n61 = Variant To Data(error in=w313, type="Light Property", Variant=w312) -> (data=w307:T5, error out=w305:errorcluster)
              n62 = Variant To Data(error in=w345, type="Axis Property", Variant=w344) -> (data=w340:T7, error out=w339:errorcluster)
              n63 = Variant To Data(error in=w335, type="Value Pair Property", Variant=w336) -> (data=w330:T14, error out=w331:errorcluster)
              n64 = Variant To Data(error in=w303, type="Format Property", Variant=w302) -> (data=w298:T16, error out=w297:errorcluster)
              n65 = Variant To Data(error in=w325, type="Cursor Property Array", Variant=w324) -> (data=w322:T17, error out=w329:errorcluster)
              n66 = Variant To Data(error in=w319, type="3D Bar Property Array", Variant=w320) -> (data=w287:T26, error out=w316:errorcluster)
              n67 = Bundle By Name(cluster=w288, "3D Bar Property Array"=w287) -> (w286:refnum<class "3D Bar.lvclass">)
              n68 = Bundle By Name(cluster=w355, "Graph Property"=w308, "Light Property"=w307, "Axis Property"=w340, "Value Pair Property"=w330, "Format Property"=w298, "Cursor Property Array"=w322) -> (w354:T32)
            }
          }
        }
      }
      event "Page List": Value Change {
        n69 = event-data() -> ("NewVal"=w356:i32)  [unwired: 1 out]
        n70 = case shown="0, Default" w356 {
          tunnel: w363 -> [w376 _ _ _ _ _ _]
          tunnel: [w376 w377 w378 w379 w380 w381 w382] -> w364
          tunnel: w362 -> [_ w377 _ _ _ _ _]
          tunnel: w361 -> [_ _ w378 _ _ _ _]
          tunnel: w360 -> [_ _ _ w379 _ _ _]
          tunnel: w359 -> [_ _ _ _ w380 _ _]
          tunnel: w358 -> [_ _ _ _ _ w381 _]
          tunnel: w357 -> [_ _ _ _ _ _ w382]
          frame 0, Default {
          }
          frame 1 {
          }
          frame 2 {
          }
          frame 3 {
          }
          frame 4 {
          }
          frame 5 {
          }
          frame 6 {
          }
        }
        n71 = invoke on="Bar Panel" class="SubPnl" method="Insert VI"("VI Ref"=w364) -> ()  [unwired: 3 in, 4 out]
      }
      event "Cancel": Value Change; Panel Close {
        w383 = TRUE
        n72 = event-data() -> ()  [unwired: 4 out]
        n73 = invoke class="VI" method="Abort VI"(reference=w396, error in=w397) -> (reference out=w394:refnum<vi>, error out=w395:errorcluster)  [unwired: 1 in, 1 out]
        n74 = invoke class="VI" method="Abort VI"(reference=w401, error in=w400) -> (reference out=w398:refnum<vi>, error out=w399:errorcluster)  [unwired: 1 in, 1 out]
        n75 = invoke class="VI" method="Abort VI"(reference=w411, error in=w413) -> (reference out=w410:refnum<vi>, error out=w412:errorcluster)  [unwired: 1 in, 1 out]
        n76 = invoke class="VI" method="Abort VI"(reference=w407, error in=w409) -> (reference out=w406:refnum<vi>, error out=w408:errorcluster)  [unwired: 1 in, 1 out]
        n77 = invoke class="VI" method="Abort VI"(reference=w403, error in=w405) -> (reference out=w402:refnum<vi>, error out=w404:errorcluster)  [unwired: 1 in, 1 out]
        n78 = invoke class="VI" method="Abort VI"(reference=w393, error in=w392) -> (reference out=w385:refnum<vi>, error out=w386:errorcluster)  [unwired: 1 in, 1 out]
        n79 = invoke class="VI" method="Abort VI"(reference=w391, error in=w390) -> (reference out=w388:refnum<vi>, error out=w387:errorcluster)  [unwired: 1 in, 1 out]
      }
      event "Help": Value Change {
        n80 = event-data() -> ()  [unwired: 7 out]
        n81 = local read "Page List"() -> (w416:i32)
        n82 = case shown="0, Default" w416 {
          tunnel: w424 -> [w441 _ _ _ _ _ _]
          tunnel: [w441 w442 w443 w444 w445 w446 w447] -> w423
          tunnel: w422 -> [_ w442 _ _ _ _ _]
          tunnel: w421 -> [_ _ w443 _ _ _ _]
          tunnel: w420 -> [_ _ _ w444 _ _ _]
          tunnel: w419 -> [_ _ _ _ w445 _ _]
          tunnel: w418 -> [_ _ _ _ _ w446 _]
          tunnel: w417 -> [_ _ _ _ _ _ w447]
          frame 0, Default {
          }
          frame 1 {
          }
          frame 2 {
          }
          frame 3 {
          }
          frame 4 {
          }
          frame 5 {
          }
          frame 6 {
          }
        }
        n83 = property class="VI"(reference=w423) -> (error out=w426:errorcluster, "Help.Tag"=w428:string, "Help.Path"=w429:path)  [unwired: 1 in, 1 out]
        n84 = Strip Path(path=w429) -> (name=w427:string)  [unwired: 1 out]
        n85 = call <helpdir>:"_LaunchHelp.vi"("error in (no error)"=w426, "CHM or HLP filename (lvdialog.chm)"=w427, "HTML filename"=w428) -> ("error out"=w425:errorcluster)  [unwired: 4 out]
        n86 = call <vilib>:"Clear Errors.vi"("error in (no error)"=w425) -> ()  [unwired: 5 in, 2 out]
      }
    }
  }
  "Cancel?" <- w79
  n87 = Close Reference(reference=w112, error in (no error)=w9) -> (error out=w87:errorcluster)
  n88 = Close Reference(reference=w63, error in (no error)=w8) -> (error out=w61:errorcluster)
  n89 = Close Reference(reference=w105, error in (no error)=w7) -> (error out=w62:errorcluster)
  n90 = Close Reference(reference=w100, error in (no error)=w6) -> (error out=w14:errorcluster)
  n91 = Close Reference(reference=w53, error in (no error)=w5) -> (error out=w13:errorcluster)
  n92 = Close Reference(reference=w95, error in (no error)=w4) -> (error out=w12:errorcluster)
  n93 = Close Reference(reference=w90, error in (no error)=w3) -> (error out=w11:errorcluster)
  n94 = Unregister For Events(event registration refnum=w30, error in=w32) -> (error out=w33:errorcluster)
  n95 = Destroy User Event(user event=w31, error in=w33) -> (error out=w10:errorcluster)
  n96 = Merge Errors(w87, w61, w62, w14, w13, w12, w11, w10) -> (w2:errorcluster)
  n97 = invoke on="Bar Panel" class="SubPnl" method="Remove VI"(error in=w2) -> (error out=w1:errorcluster)  [unwired: 2 in, 2 out]
  n98 = call <vilib>:"Write Property.vi"("error in (no error)"=w1, "Property Cluster"=w116, "3D Plot.lvclass in"=w88) -> ("error out"=w39:errorcluster, "3D Plot.lvclass out"=→"3D Bar out":refnum<class "3D Bar.lvclass">)  [unwired: 7 out]
  n99 = call <vilib>:"Temp Scene Update.vi"("State"=Temp_Scene_State."Destory", "error in (no error)"=w39) -> ("error out"=→"error out":errorcluster)  [unwired: 4 in, 5 out]
  "Object Cluster Out" <- "Object Cluster In"
